vi "Packer. 1-I16 As U64.vi"(8 "Input Valid":bool, 9 "flush":bool, 10 "data":i16) -> (0 "Output Valid":bool, 1 "byteEnables":u16=255 format="%.0x", 2 "i16 as u64":u64)   [LabVIEW 2011]
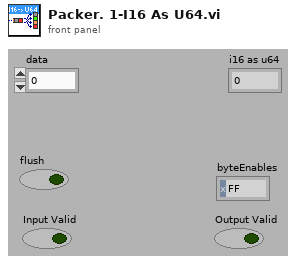
[diagram p1: front panel]
types:
  T1 = cluster{"i 1":i16, "i 2":i16, "i 3":i16, "i 4":i16}
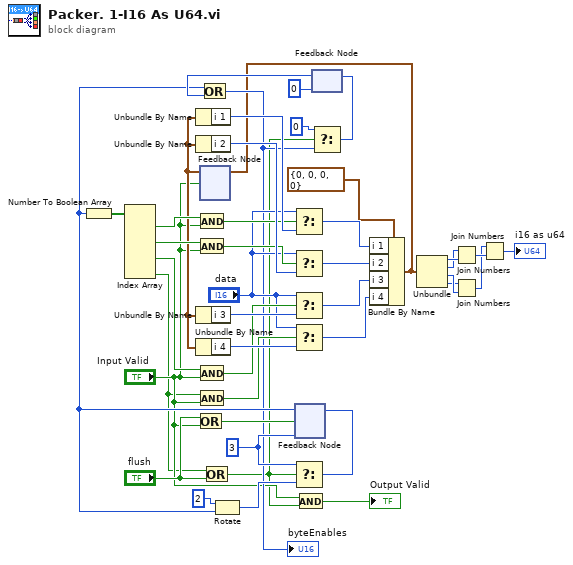
[diagram p0: block diagram]
diagram:
  w20 = u16 3
  n1 = Or(x="flush", y="Input Valid") -> (x .or. y?=w23:bool)
  n2 = feedback #1() -> (w10:T1)  [unwired: 1 in]
  n3 = Unbundle By Name(w10) -> ("i 1"=w41:i16)
  n4 = Unbundle By Name(w10) -> ("i 2"=w40:i16)
  n5 = Unbundle By Name(w10) -> ("i 3"=w39:i16)
  n6 = Unbundle By Name(w10) -> ("i 4"=w38:i16)
  n7 = feedback #2(w20) -> (w19:u16)
  n8 = Number To Boolean Array(number=w19) -> (Boolean array=w11:bool[])
  n9 = Index Array(array=w11) -> (element #1=w31:bool, element #3=w30:bool, element #5=w29:bool, element #7=w8:bool)  [unwired: 7 in, 3 out]
  n10 = And(x=w31, y="Input Valid") -> (x .and. y?=w35:bool)
  n11 = And(x=w30, y="Input Valid") -> (x .and. y?=w34:bool)
  n12 = And(x=w29, y="Input Valid") -> (x .and. y?=w33:bool)
  n13 = And(x=w8, y="Input Valid") -> (x .and. y?=w32:bool)
  n14 = Or(x=w8, y="flush") -> (x .or. y?=w7:bool)
  n15 = Rotate(1:w19, 2:u16 2 ("y")) -> (0:w22:u16)
  n16 = Select(t="data", s=w35, f=w41) -> (s? t:f=w43:i16)
  n17 = Select(t="data", s=w34, f=w40) -> (s? t:f=w42:i16)
  n18 = Select(t="data", s=w33, f=w39) -> (s? t:f=w37:i16)
  n19 = Select(t="data", s=w32, f=w38) -> (s? t:f=w36:i16)
  n20 = Select(t=w20, s=w7, f=w22) -> (s? t:f=w21:u16)
  n21 = feedback-in #2(w21, w23) -> ()
  n22 = And(x="Input Valid", y=w7) -> (x .and. y?=→"Output Valid":bool)
  n23 = feedback #3(u16 0) -> (w27:u16)
  n24 = Or(x=w19, y=w27) -> (x .or. y?=w15:u16)
  "byteEnables" <- w15
  n25 = Select(t=u16 0, s=w7, f=w15) -> (s? t:f=w24:u16)
  n26 = feedback-in #3(w24) -> ()
  n27 = Bundle By Name(cluster=T1 {"i 1"=0, "i 2"=0, "i 3"=0, "i 4"=0}, "i 1"=w43, "i 2"=w42, "i 3"=w37, "i 4"=w36) -> (w13:T1)
  n28 = feedback-in #1(w13, "Input Valid") -> ()
  n29 = Unbundle(w13) -> ("i 1"=w6:i16, "i 2"=w5:i16, "i 3"=w4:i16, "i 4"=w3:i16)
  n30 = Join Numbers(hi=w5, lo=w6) -> ((hi.lo)=w2:u32)
  n31 = Join Numbers(hi=w3, lo=w4) -> ((hi.lo)=w1:u32)
  n32 = Join Numbers(hi=w1, lo=w2) -> ((hi.lo)=→"i16 as u64":u64)
